vi "GmailLV80.vi"(4 "Body":string="LabVIEW is the coolest!!!", 5 "Subject":string="Gmail Thru LabVIEW!!!", 6 "Recipient's Email Address":string, 7 "Sender's Email Address (eg: LabVIEW@gmail.com)":string="jbowles.irm@gmail.com", 8 "Port":i32=587, 9 "GMAIL Account Password":string, 10 "GMAIL Account User ID":string="jbowles.irm", 11 "Outgoing Mail Server (SMTP)":string="smtp.gmail.com") -> ()   [LabVIEW 2009]
panel:
  in  "CC - Optional":string
  in  "Attachment - Optional":path
  in  "Enable SSL":bool=TRUE
  in  "Recipient's Name":string
  in  "Sender's Name":string
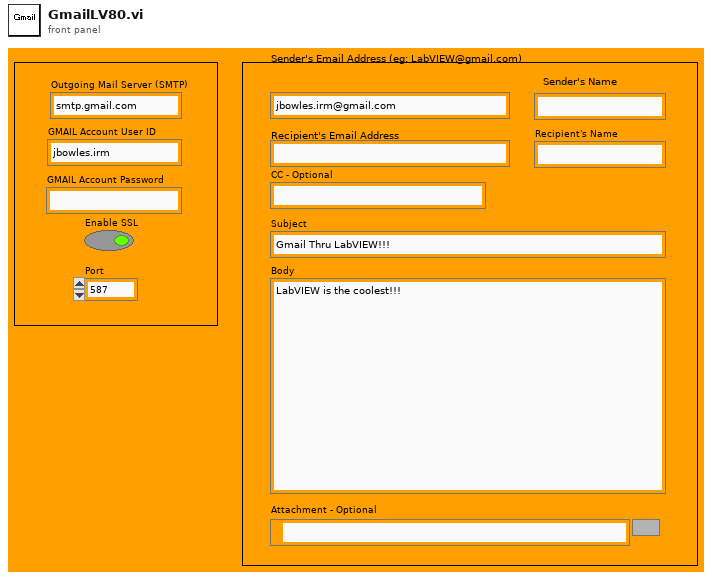
[diagram p1: front panel]
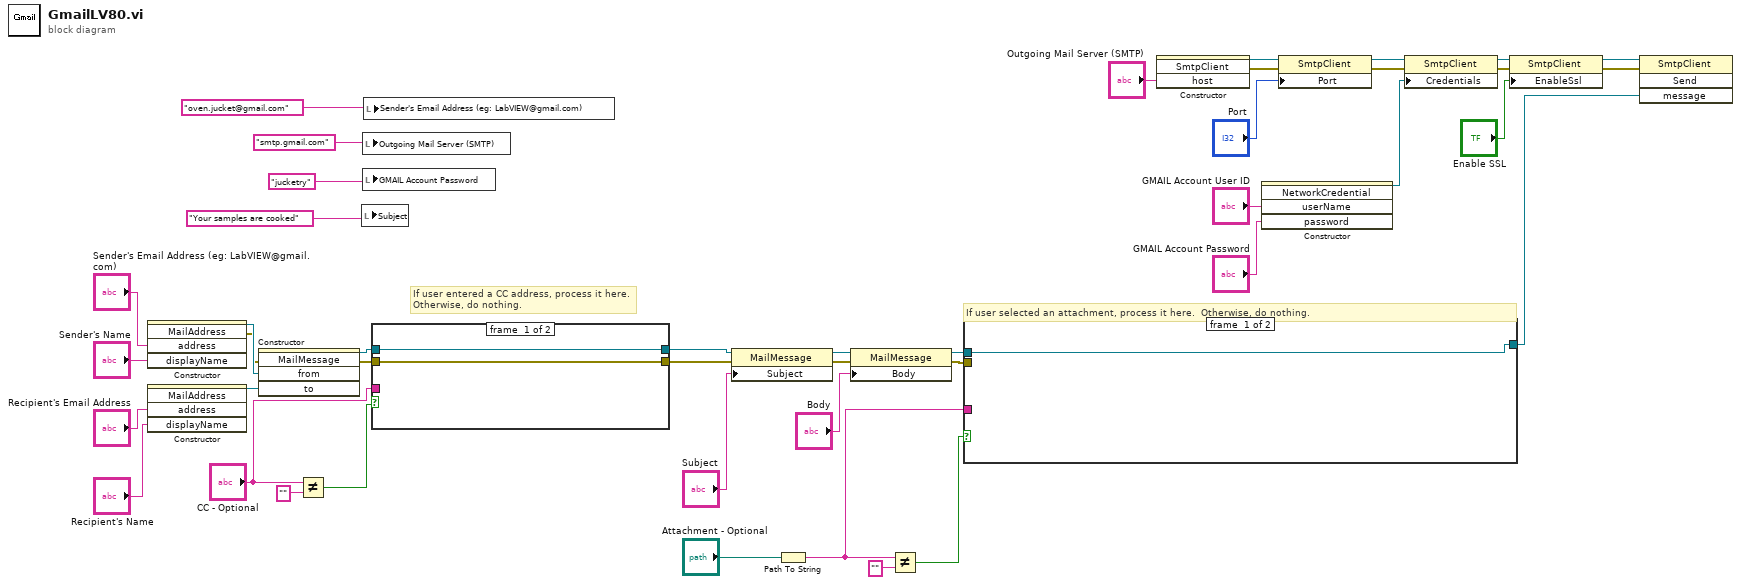
[diagram p0: block diagram]
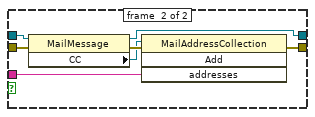
[diagram p2: hidden frame]
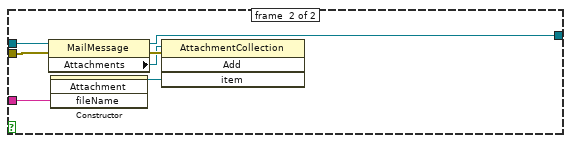
[diagram p3: hidden frame]
diagram:
  # "If user selected an attachment, process it here.  Otherwise, do nothing."
  # "If user entered a CC address, process it here.\nOtherwise, do nothing."
  n1 = constructor class="MailAddress"("address"="Sender's Email Address (eg: LabVIEW@gmail.com)", "displayName"="Sender's Name") -> (reference out=w42:refnum<k24>, error out=w6:errorcluster)  [unwired: 3 in, 3 out]
  n2 = constructor class="MailAddress"("address"="Recipient's Email Address", "displayName"="Recipient's Name") -> (reference out=w43:refnum<k24>)  [unwired: 3 in, 4 out]
  n3 = constructor class="MailMessage"(error in=w6, "from"=w42, "to"=w43) -> (reference out=w13:refnum<k24>, error out=w12:errorcluster)  [unwired: 2 in, 3 out]
  n4 = Not Equal?(x="CC - Optional", y="") -> (x != y?=w15:bool)
  n5 = local write "Subject"("Your samples are cooked") -> ()
  n6 = local write "Outgoing Mail Server (SMTP)"("smtp.gmail.com") -> ()
  n7 = local write "GMAIL Account Password"("jucketry") -> ()
  n8 = local write "Sender's Email Address (eg: LabVIEW@gmail.com)"("oven.jucket@gmail.com") -> ()
  n9 = case shown="True" w15 {
    tunnel: "CC - Optional" -> [_ w50]
    tunnel: w13 -> [w45 w49]
    tunnel: w12 -> [w44 w48]
    tunnel: [w45 w47] -> w11
    tunnel: [w44 w46] -> w10
    frame #0 {
    }
    frame #1 {
      n10 = property class="MailMessage"(reference=w49, error in=w48) -> (reference out=w47:refnum<k24>, error out=w52:errorcluster, "CC"=w51:refnum<k24>)
      n11 = invoke class="MailAddressCollection" method="Add"(reference=w51, error in=w52, "addresses"=w50) -> (error out=w46:errorcluster)  [unwired: 1 in, 3 out]
    }
  }
  n12 = property class="MailMessage"(reference=w11, error in=w10, "Subject"="Subject") -> (reference out=w33:refnum<k24>, error out=w41:errorcluster)
  n13 = Path To String(path="Attachment - Optional") -> (string=w17:string)
  n14 = property class="MailMessage"(reference=w33, error in=w41, "Body"="Body") -> (reference out=w21:refnum<k24>, error out=w5:errorcluster)
  n15 = Not Equal?(x=w17, y="") -> (x != y?=w18:bool)
  n16 = case shown="True" w18 {
    tunnel: w21 -> [w53 w57]
    tunnel: [w53 w56] -> w9
    tunnel: w17 -> [_ w55]
    tunnel: w5 -> [_ w54]
    frame #0 {
    }
    frame #1 {
      n17 = property class="MailMessage"(reference=w57, error in=w54) -> (reference out=w56:refnum<k24>, error out=w60:errorcluster, "Attachments"=w58:refnum<k24>)
      n18 = constructor class="Attachment"("fileName"=w55) -> (reference out=w59:refnum<k24>)  [unwired: 3 in, 3 out]
      n19 = invoke class="AttachmentCollection" method="Add"(reference=w58, error in=w60, "item"=w59) -> ()  [unwired: 1 in, 4 out]
    }
  }
  n20 = constructor class="SmtpClient"("host"="Outgoing Mail Server (SMTP)") -> (reference out=w27:refnum<k24>, error out=w24:errorcluster)  [unwired: 3 in, 2 out]
  n21 = constructor class="NetworkCredential"("userName"="GMAIL Account User ID", "password"="GMAIL Account Password") -> (reference out=w28:refnum<k24>)  [unwired: 3 in, 4 out]
  n22 = property class="SmtpClient"(reference=w27, error in=w24, "Port"="Port") -> (reference out=w26:refnum<k24>, error out=w23:errorcluster)
  n23 = property class="SmtpClient"(reference=w26, error in=w23, "Credentials"=w28) -> (reference out=w25:refnum<k24>, error out=w22:errorcluster)
  n24 = property class="SmtpClient"(reference=w25, error in=w22, "EnableSsl"="Enable SSL") -> (reference out=w7:refnum<k24>, error out=w8:errorcluster)
  n25 = invoke class="SmtpClient" method="Send"(reference=w7, error in=w8, "message"=w9) -> ()  [unwired: 1 in, 4 out]
